vi "Main.vi"() -> ()   [LabVIEW 2018]
uses:
  Open_device_2017.llb/Select_Instr.ctl
  Stany.ctl
  <vilib>/express/express shared/transition.llb/Dynamic To Waveform Array.vi
  <vilib>/express/express signal manip/GetorSetDDTAttributes/Set DDT Attributes/SetT0.vi
  <vilib>/express/express shared/transition.llb/Waveform Array To Dynamic.vi
  <vilib>/express/express signal manip/GetorSetDDTAttributes/Set DDT Attributes/Set DDT Properties.xnode
panel:
  in  "Narysuj":bool
  out "Tablica transmitancji":dbl[](array[numeric])
  out "Tablica częstotliwości":dbl[](array[numeric])
  out "Gęstość-1":dbl
  out "Charakterystyka częstotliwościowa czwórnika":T1(graph)
  in  "Tabela danych pomiarowych":string[][](table)
  in  "Rozłożenie":bool
  in  "Gęstość":dbl=20.0 min=3.0 max=1000.0
  in  "Częstotliwość początkowa":dbl=10.0 min=0.1 max=15000000.0 format="%.1f"
  in  "Amplituda":dbl=5.0 min=0.05 max=10.0 format="%.2f"
  in  "Częstotliwość końcowa":dbl=10000.0 min=0.1 max=15000000.0 format="%.1f"
  out "Linia błędów":errorcluster
  in  "Stop":bool
  in  "Przerwij":bool
  in  "Zapis":bool
  in  "Pomiar":bool
  # "Dane wejściowe"
  # "Dane wejściowe"
  # "Ustawienia generatora"
  # "Hz"
  # "Hz"
  # "V"
  # "Konfiguracja punktów pomiarowych"
  # "punktów"
  # "LIN"
  # "LOG"
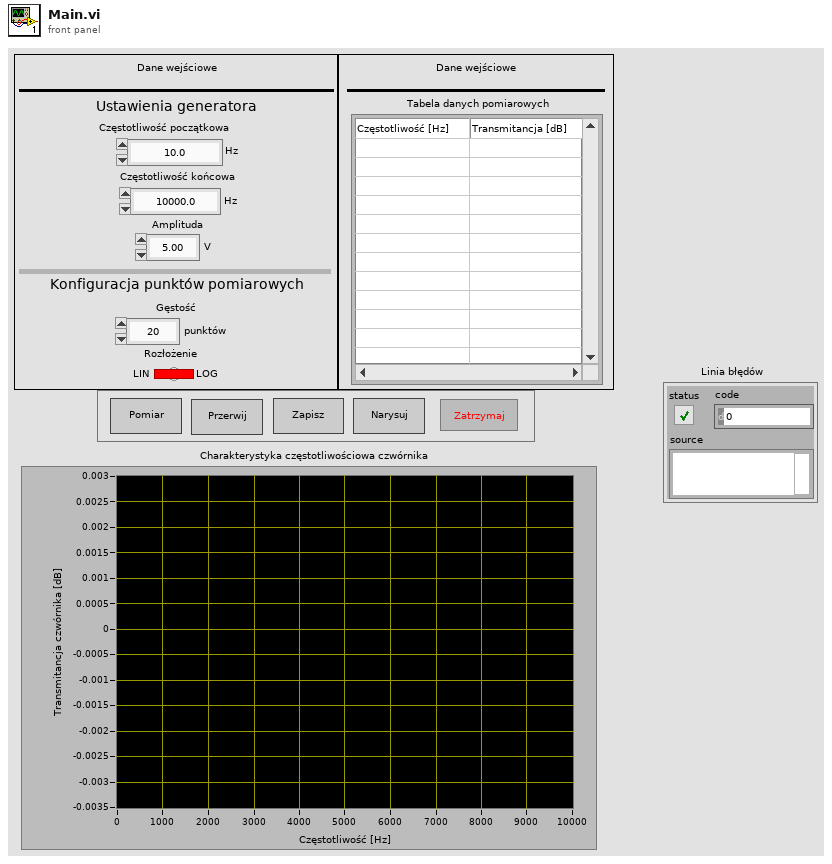
[diagram p1: front panel]
types:
  T1 = cluster{"Tablica częstotliwości":dbl[], "Losowa tablica":dbl[]}
  T2 = typedef "Select_Instr.ctl" = string
  T3 = cluster{"VISA resource name 1":refnum<visa-resource-name>, "VISA resource name 2":refnum<visa-resource-name>}
  T4 = typedef "Stany.ctl" = enum16{"Idle", "Inicjalizacja", "Pomiar", "Zapis", "Narysuj"}
  T5 = enum8{"Enabled", "Disabled", "Disabled and Grayed Out"}
  T6 = cluster{"Tablica częstotliwości":dbl[], "Tablica transmitancji":dbl[]}
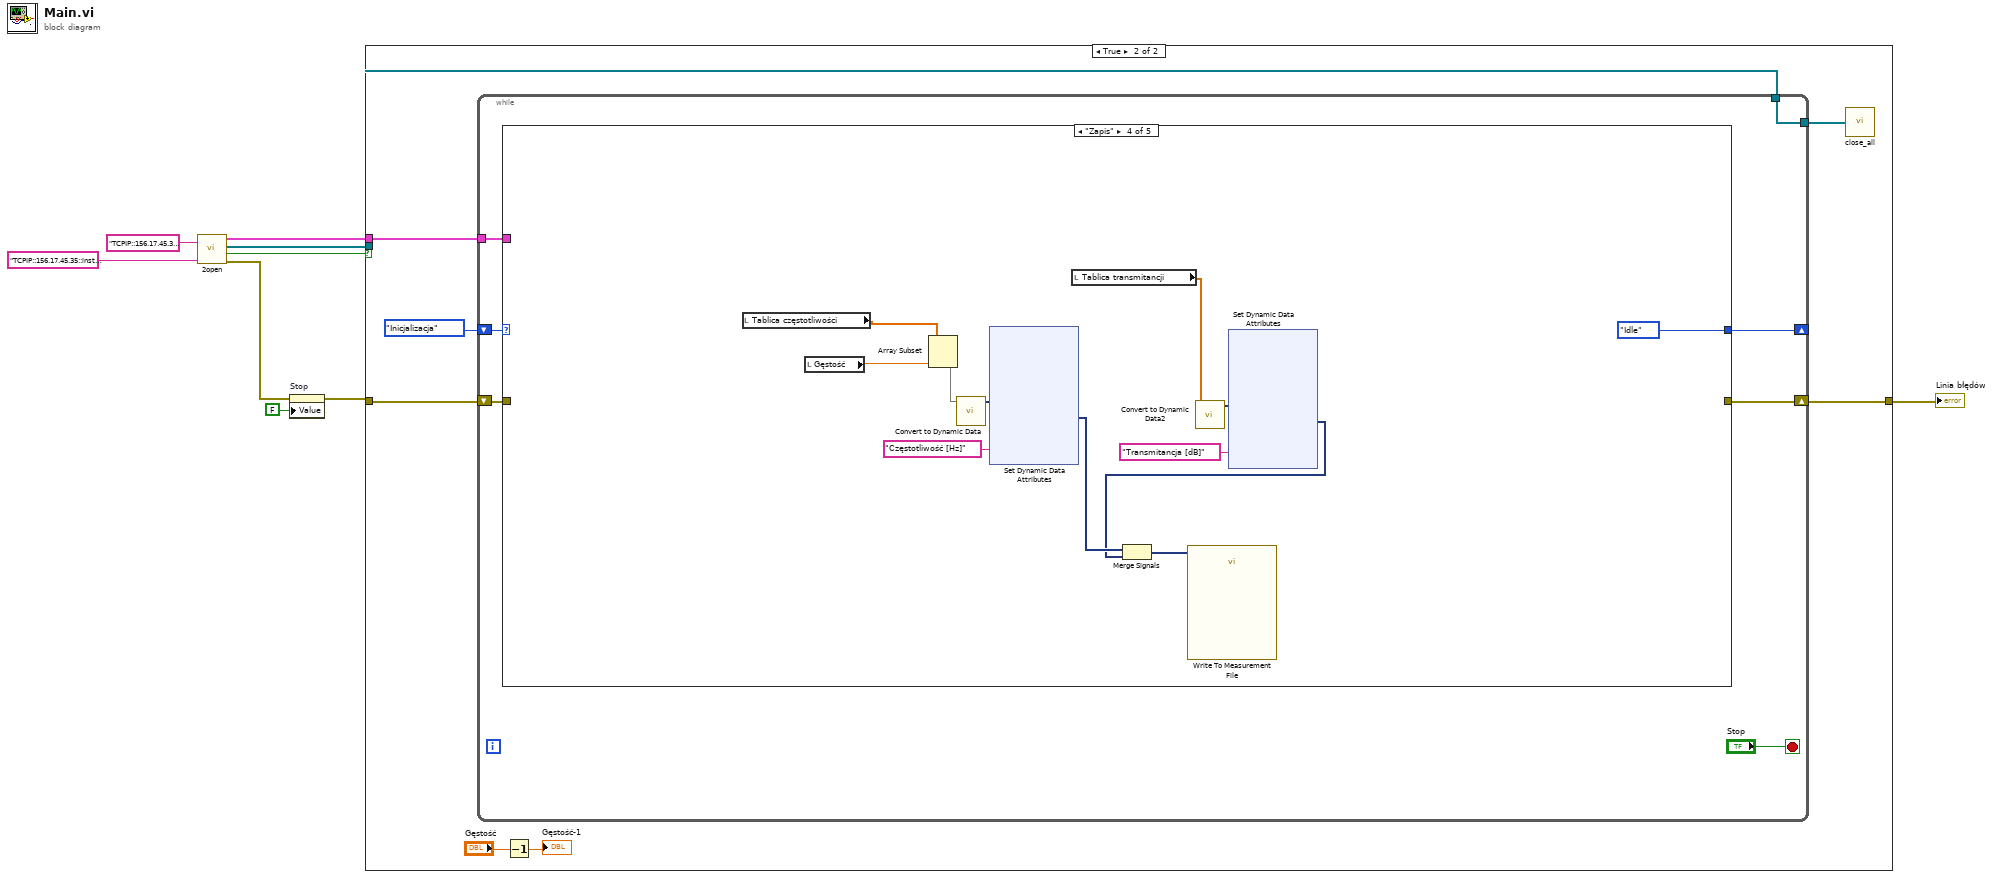
[diagram p0: block diagram]
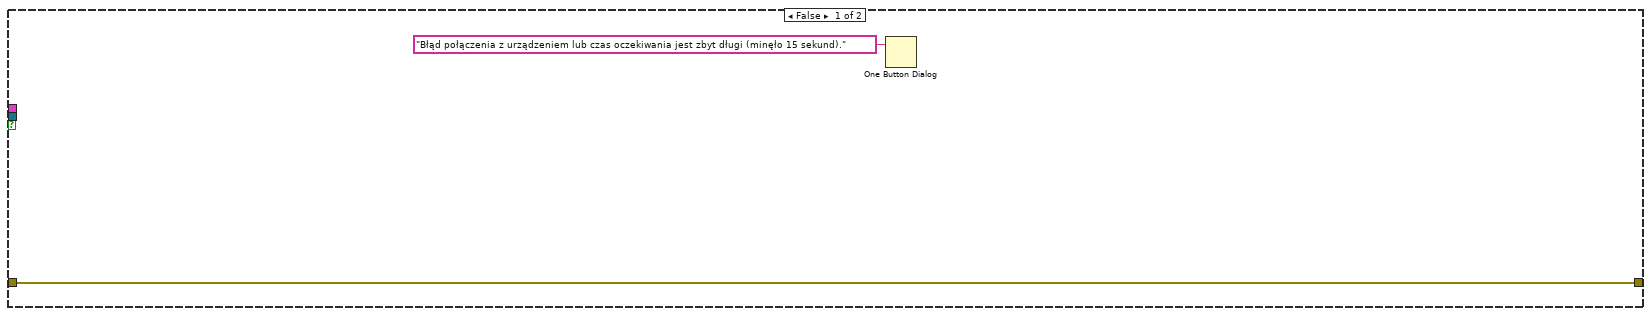
[diagram p2: hidden frame]
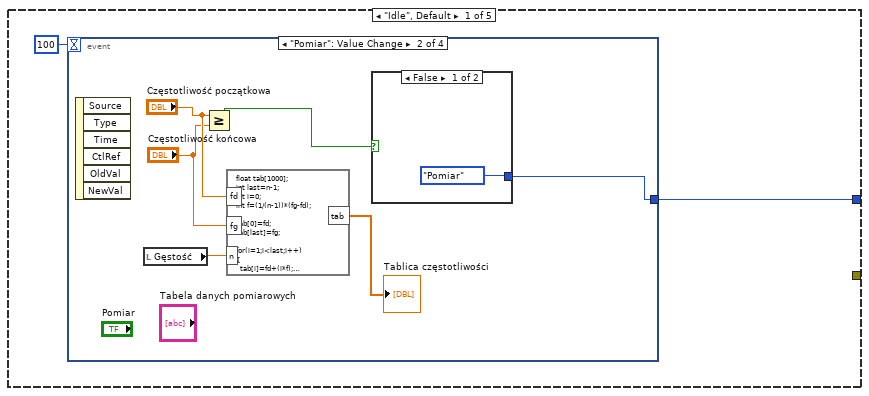
[diagram p3: hidden frame]
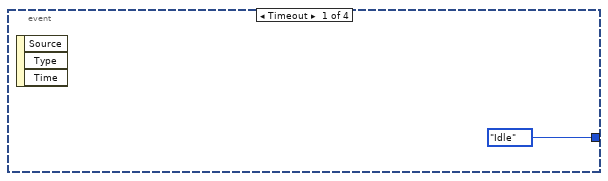
[diagram p4: hidden frame]
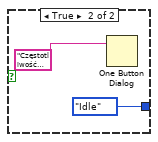
[diagram p5: hidden frame]
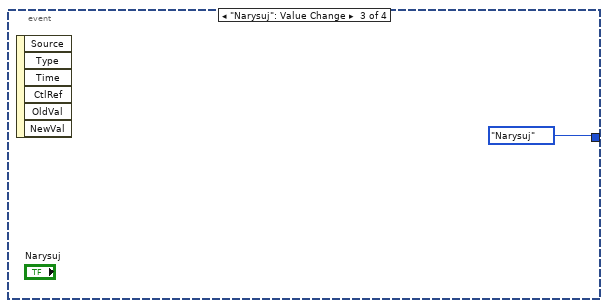
[diagram p6: hidden frame]
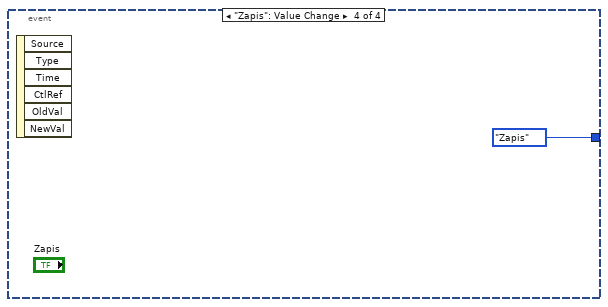
[diagram p7: hidden frame]
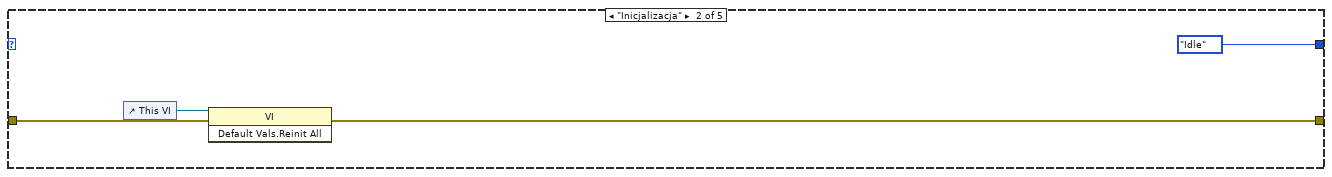
[diagram p8: hidden frame]
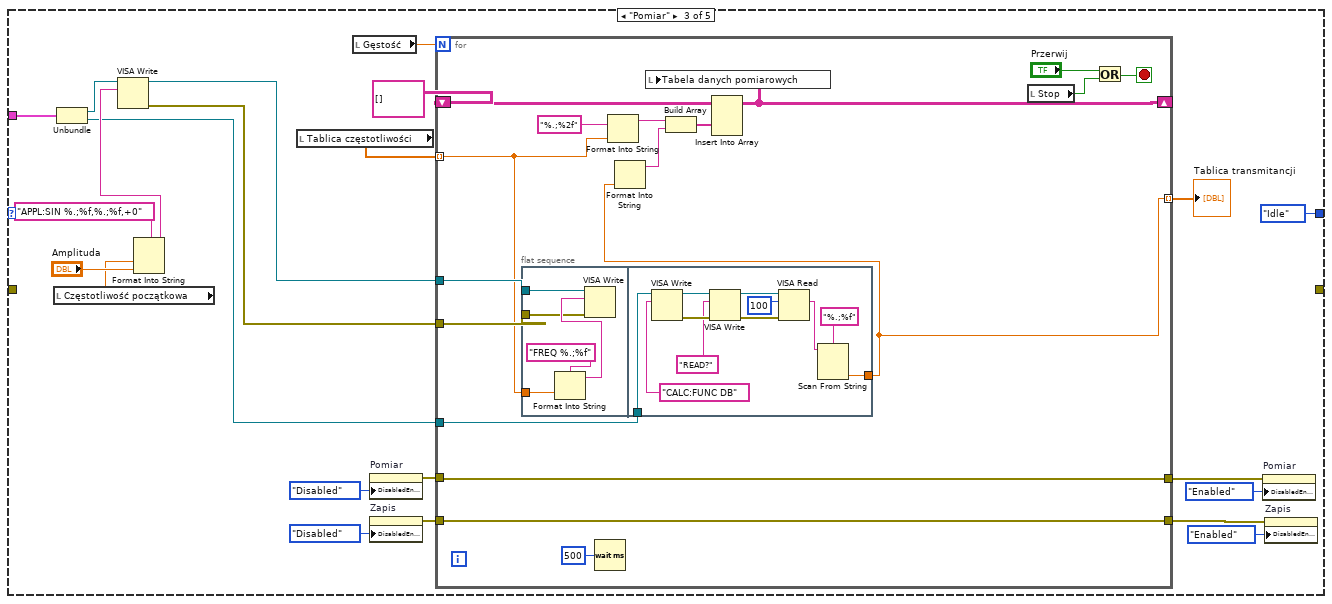
[diagram p9: hidden frame]
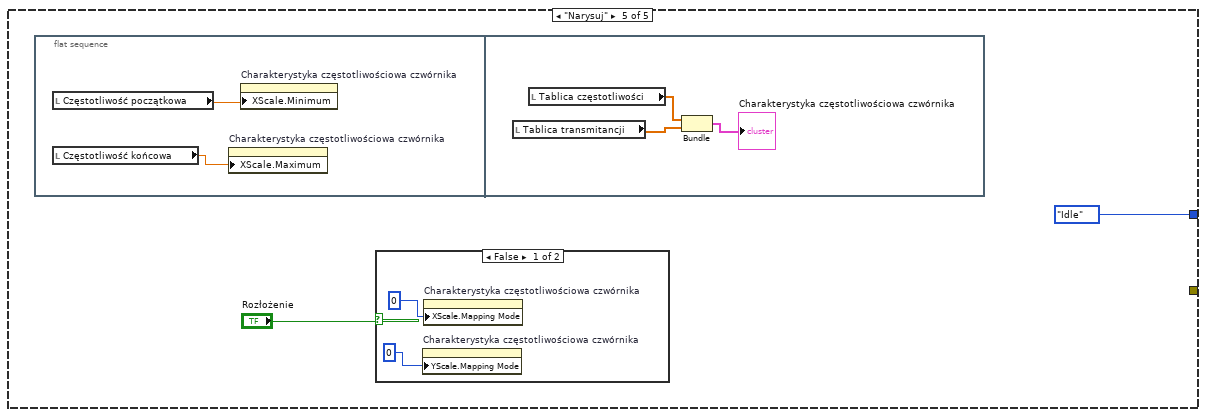
[diagram p10: hidden frame]
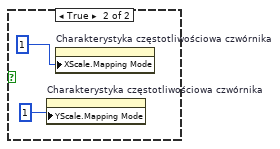
[diagram p11: hidden frame]
diagram:
  n1 = call "2open.vi"("VISA resource name 1"=T2 "TCPIP::156.17.45.35::inst3::INSTR" ("Select_Instrument"), "VISA resource name 2"=T2 "TCPIP::156.17.45.35::inst5::INSTR" ("Select_Instrument")) -> ("InstrCluster"=w4:T3, "InstrArray"=w5:refnum<visa-resource-name>[], "Open OK (true)"=w3:bool, "error out"=w6:errorcluster)
  n2 = property on="Stop" class="Bool (strict)"(error in=w6, "Value"=FALSE ("Stop")) -> (error out=w9:errorcluster)  [unwired: 1 in, 1 out]
  n3 = case shown="True" w3 {
    tunnel: w4 -> [_ w19]
    tunnel: w5 -> [_ w18]
    tunnel: w9 -> [w11 w17]
    tunnel: [w11 w14] -> w7
    frame False {
      n4 = One Button Dialog(message="Błąd połączenia z urządzeniem lub czas oczekiwania jest zbyt długi (minęło 15 sekund).") -> ()  [unwired: 1 in, 1 out]
    }
    frame True {
      n5 = while {
        tunnel: w18 -> [w25]
        tunnel: [w25] -> w16
        shift-right: [w21] -> w14
        shift-left: w17 -> [w22]
        tunnel: w19 -> [w26]
        shift-right: [w23] -> _
        shift-left: Stany."Inicjalizacja" -> [w24]
        stop <- "Stop" stop-if-true
        n6 = case shown="\"Zapis\"" w24 {
          tunnel: w26 -> [_ _ w53 _ _]
          tunnel: [w27 Stany."Idle" Stany."Idle" Stany."Idle" Stany."Idle"] -> w23
          tunnel: w22 -> [_ w42 _ _ _]
          tunnel: [_ w41 _ _ _] -> w21
          frame "Idle", Default {
            n7 = event shown="[1] \"Pomiar\": Value Change" {
              selector: _ -> [_ _ _ _]
              dyn-events: _ -> [_ _ _ _]
              timeout: 100 -> [_ _ _ _]
              tunnel: [Stany."Idle" w30 Stany."Narysuj" Stany."Zapis"] -> w27
              event Timeout {
                n8 = event-data() -> ()  [unwired: 1 in, 3 out]
              }
              event "Pomiar": Value Change {
                n9 = event-data() -> ()  [unwired: 1 in, 6 out]
                n10 = local read "Gęstość"() -> (w35:dbl)
                n11 = Greater Or Equal?(x="Częstotliwość początkowa", y="Częstotliwość końcowa") -> (x >= y?=w32:bool)
                n12 = formula code="float tab[1000];\nint last=n-1;\nint i=0;\nint f=(1/(n-1))*(fg-fd);\n\ntab[0]=fd;\ntab[last]=fg;\n\nfor(i=1;i<last;i++)\n{\n  tab[i]=fd+(i*f);\n}"("fd"="Częstotliwość początkowa", "fg"="Częstotliwość końcowa", "n"=w35) -> ("tab"=→"Tablica częstotliwości":dbl[])
                n13 = case shown="False" w32 {
                  tunnel: [Stany."Pomiar" Stany."Idle"] -> w30
                  frame False {
                  }
                  frame True {
                    n14 = One Button Dialog(message="Częstotliwość początkowa musi być mniejsza niż częstotliwość końcowa.") -> ()  [unwired: 1 in, 1 out]
                  }
                }
              }
              event "Narysuj": Value Change {
                n15 = event-data() -> ()  [unwired: 1 in, 6 out]
              }
              event "Zapis": Value Change {
                n16 = event-data() -> ()  [unwired: 1 in, 6 out]
              }
            }
          }
          frame "Inicjalizacja" {
            n17 = control-ref of="This VI"() -> (w43:refnum<vi>)
            n18 = invoke class="VI" method="Default Vals.Reinit All"(reference=w43, error in=w42) -> (error out=w41:errorcluster)  [unwired: 1 in, 2 out]
          }
          frame "Pomiar" {
            n19 = local read "Częstotliwość początkowa"() -> (w50:dbl)
            n20 = Unbundle(w53) -> ("VISA resource name 1"=w52:refnum<visa-resource-name>, "VISA resource name 2"=w47:refnum<visa-resource-name>)
            n21 = Format Into String(format string="APPL:SIN %.;%f,%.;%f,+0" ("initial string"), w50, "Amplituda") -> (resulting string=w48:string)  [unwired: 2 in, 1 out]
            n22 = VISA Write(VISA resource name=w52, write buffer=w48) -> (VISA resource name out=w45:refnum<visa-resource-name>, error out=w46:errorcluster)  [unwired: 1 in, 1 out]
            n23 = local read "Tablica częstotliwości"() -> (w56:dbl[])
            n24 = local read "Gęstość"() -> (w57:dbl)
            n25 = property on="Pomiar" class="Bool"("DisabledEnum"=T5."Disabled" ("Disabled")) -> (error out=w65:errorcluster)  [unwired: 2 in, 1 out]
            n26 = property on="Zapis" class="Bool"("DisabledEnum"=T5."Disabled" ("Disabled")) -> (error out=w64:errorcluster)  [unwired: 2 in, 1 out]
            n27 = for {
              N: w57 -> [_]
              tunnel: w65 -> [w79]
              tunnel: w64 -> [w80]
              tunnel: [w80] -> w60
              tunnel: [w79] -> w59
              tunnel: w56 -> [w69] mode=indexing
              shift-right: [w72] -> _
              shift-left: string[][] [] -> [w73]
              tunnel: [w67] -> w54 mode=indexing
              tunnel: w47 -> [w68]
              tunnel: w46 -> [w71]
              tunnel: w45 -> [w70]
              stop <- w81 stop-if-true
              n28 = flat-sequence {
                tunnel: w71 -> [w86]
                tunnel: w70 -> [w85]
                tunnel: w69 -> [w84]
                tunnel: w68 -> [w99]
                tunnel: [w90] -> w67
                frame #0 {
                  n29 = Format Into String(format string="FREQ %.;%f", w84) -> (resulting string=w88:string)  [unwired: 2 in, 1 out]
                  n30 = VISA Write(VISA resource name=w85, write buffer=w88, error in (no error)=w86) -> ()  [unwired: 3 out]
                }
                frame #1 {
                  n31 = VISA Write(VISA resource name=w99, write buffer="CALC:FUNC DB") -> (VISA resource name out=w96:refnum<visa-resource-name>, error out=w97:errorcluster)  [unwired: 1 in, 1 out]
                  n32 = VISA Write(VISA resource name=w96, write buffer="READ?", error in (no error)=w97) -> (VISA resource name out=w93:refnum<visa-resource-name>, error out=w94:errorcluster)  [unwired: 1 out]
                  n33 = VISA Read(VISA resource name=w93, byte count=u32 100, error in (no error)=w94) -> (read buffer=w91:string)  [unwired: 3 out]
                  n34 = Scan From String(format string="%.;%f", input string=w91) -> (output 1=w90:dbl)  [unwired: 3 in, 3 out]
                }
              }
              n35 = Wait (ms)(milliseconds to wait=u32 500) -> ()  [unwired: 1 out]
              n36 = Format Into String(format string="%.;%2f" ("initial string"), w69) -> (resulting string=w75:string)  [unwired: 2 in, 1 out]
              n37 = Format Into String(w67) -> (resulting string=w78:string)  [unwired: 3 in, 1 out]
              n38 = Build Array(w75, w78) -> (w76:string[])
              n39 = Insert Into Array(array=w73, new element=w76) -> (w72:string[][])  [unwired: 2 in]
              n40 = local write "Tabela danych pomiarowych"(w72) -> ()
              n41 = local read "Stop"() -> (w82:bool)
              n42 = Or(x="Przerwij", y=w82) -> (x .or. y?=w81:bool)
            }
            "Tablica transmitancji" <- w54
            n43 = property on="Pomiar" class="Bool"(error in=w59, "DisabledEnum"=T5."Enabled" ("Disabled")) -> ()  [unwired: 1 in, 2 out]
            n44 = property on="Zapis" class="Bool"(error in=w60, "DisabledEnum"=T5."Enabled" ("Disabled")) -> ()  [unwired: 1 in, 2 out]
          }
          frame "Zapis" {
            n45 = local read "Tablica częstotliwości"() -> (w102:dbl[])
            n46 = local read "Gęstość"() -> (w103:dbl)
            n47 = Array Subset(array=w102, length=w103) -> (w110:dbl[])  [unwired: 1 in]
            n48 = call "Convert to Dynamic Data"("Array"=w110) -> ("Dynamic Data Type"=w106:dynamicdata)  [unwired: 3 in]
            n49 = xnode "Set Dynamic Data Attributes"("Signals In"=w106, "Signal Name"="Częstotliwość [Hz]") -> ("Signals Out"=w108:dynamicdata)  [unwired: 2 in, 1 out]
            n50 = local read "Tablica transmitancji"() -> (w101:dbl[])
            n51 = call "Convert to Dynamic Data2"("Array"=w101) -> ("Dynamic Data Type"=w107:dynamicdata)  [unwired: 3 in]
            n52 = xnode "Set Dynamic Data Attributes"("Signals In"=w107, "Signal Name"="Transmitancja [dB]") -> ("Signals Out"=w100:dynamicdata)  [unwired: 2 in, 1 out]
            n53 = Merge Signals(w108, w100) -> (w109:dynamicdata)
            n54 = call "Write To Measurement File"("Signals"=w109) -> ()  [unwired: 16 in, 3 out]
          }
          frame "Narysuj" {
            n55 = flat-sequence {
              frame #0 {
                n56 = local read "Częstotliwość początkowa"() -> (w146:dbl)
                n57 = local read "Częstotliwość końcowa"() -> (w147:dbl)
                n58 = property on="Charakterystyka częstotliwościowa czwórnika" class="XYGraph (strict)"("XScale.Maximum"=w147) -> ()  [unwired: 2 in, 2 out]
                n59 = property on="Charakterystyka częstotliwościowa czwórnika" class="XYGraph (strict)"("XScale.Minimum"=w146) -> ()  [unwired: 2 in, 2 out]
              }
              frame #1 {
                n60 = local read "Tablica transmitancji"() -> (w148:dbl[])
                n61 = local read "Tablica częstotliwości"() -> (w150:dbl[])
                n62 = Bundle("Tablica częstotliwości"=w150, "Tablica transmitancji"=w148) -> (→"Charakterystyka częstotliwościowa czwórnika":T6)  [unwired: 1 in]
              }
            }
            n63 = case shown="False" "Rozłożenie" {
              frame False {
                n64 = property on="Charakterystyka częstotliwościowa czwórnika" class="XYGraph (strict)"("YScale.Mapping Mode"=u8 0 ("Y Scale.Mapping Mode")) -> ()  [unwired: 2 in, 2 out]
                n65 = property on="Charakterystyka częstotliwościowa czwórnika" class="XYGraph (strict)"("XScale.Mapping Mode"=u8 0 ("X Scale.Mapping Mode")) -> ()  [unwired: 2 in, 2 out]
              }
              frame True {
                n66 = property on="Charakterystyka częstotliwościowa czwórnika" class="XYGraph (strict)"("YScale.Mapping Mode"=u8 1 ("X Scale.Mapping Mode")) -> ()  [unwired: 2 in, 2 out]
                n67 = property on="Charakterystyka częstotliwościowa czwórnika" class="XYGraph (strict)"("XScale.Mapping Mode"=u8 1 ("X Scale.Mapping Mode")) -> ()  [unwired: 2 in, 2 out]
              }
            }
          }
        }
      }
      n68 = Decrement(x="Gęstość") -> (x-1=→"Gęstość-1":dbl)
      n69 = call "close_all.vi"("OpenRes"=w16) -> ()  [unwired: 1 out]
    }
  }
  "Linia błędów" <- w7
